vi "Send and Clear Error.vi"(8 "error in (no error)":errorcluster, 11 "Dynamic Combobox in":refnum<class "Dynamic Combobox.lvclass">) -> (0 "error out":errorcluster, 3 "Dynamic Combobox out":refnum<class "Dynamic Combobox.lvclass">)   [LabVIEW 2020, in "Dynamic Combobox.lvlib" / "Dynamic Combobox.lvclass"]
uses:
  Dynamic Combobox.lvclass
  Dynamic Combobox.lvclass/Dynamic Combobox.ctl
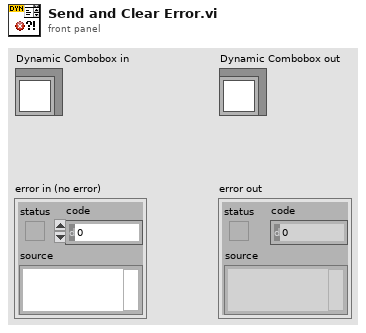
[diagram p1: front panel]
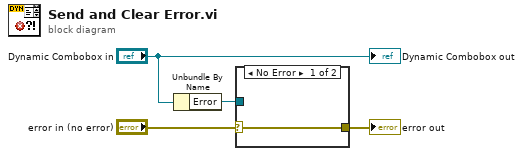
[diagram p0: block diagram]
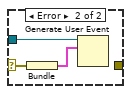
[diagram p2: hidden frame]
diagram:
  n1 = Unbundle By Name("Dynamic Combobox in") -> ("Error"=w4:refnum<user-event>)
  n2 = case shown="No Error" "error in (no error)" {
    selector: "error in (no error)" -> [w5 w7]
    tunnel: w4 -> [_ w8]
    tunnel: [w5 _] -> w1
    frame No Error {
    }
    frame Error {
      n3 = Bundle("error IO"=w7) -> (w6:cluster{"error IO":errorcluster})  [unwired: 1 in]
      n4 = Generate User Event(user event=w8, event data cluster=w6) -> ()  [unwired: 2 in, 2 out]
    }
  }
  "error out" <- w1
  "Dynamic Combobox out" <- "Dynamic Combobox in"
